vi "LeCroy.Configure Trigger.vi"(5 "Trigger Source":u16(ring) items=["Channel 1", "Channel 2", "Channel 3", "Channel 4", "External", "Line", "Ext", "Ext10"], 7 "Trigger Slope":u16(ring) items=["Rising", "Falling"], 8 "Error In":errorcluster, 10 "Trigger Level":dbl, 11 "LeCroy.Session in":T1) -> (0 "Error Out":errorcluster, 3 "LeCroy.Session out":T1)   [LabVIEW 2018]
uses:
  typedefs/LeCroy.Session.ctl
  <instrlib>/LeCroy Wave Series/Public/Configure/Configure Edge Trigger.vi
  <instrlib>/LeCroy Wave Series/LeCroy Wave Series.lvlib
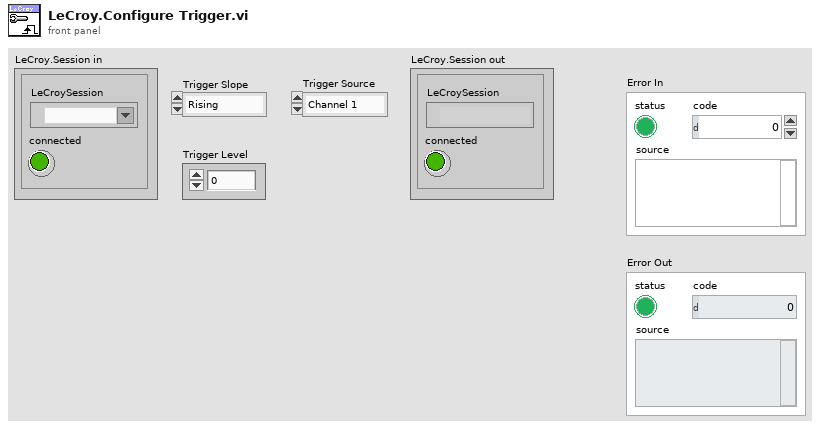
[diagram p1: front panel]
types:
  T1 = typedef "LeCroy.Session.ctl" = cluster{"LeCroySession":refnum<visa-resource-name>, "connected":bool}
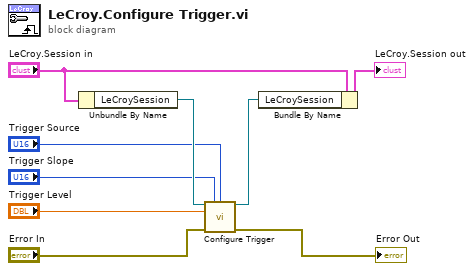
[diagram p0: block diagram]
diagram:
  n1 = Unbundle By Name("LeCroy.Session in") -> ("LeCroySession"=w9:refnum<visa-resource-name>)
  n2 = call-poly <instrlib>:"Configure Trigger.vi"("VISA resource name"=w9, "Trigger Slope (0: Rising)"="Trigger Slope", "Trigger Source (0: Channel 1)"="Trigger Source", "Trigger Level (0.0 V)"="Trigger Level", "error in (no error)"="Error In") -> ("VISA resource name out"=w8:refnum<visa-resource-name>, "error out"=→"Error Out":errorcluster)  [unwired: 9 in]
  n3 = Bundle By Name(cluster="LeCroy.Session in", "LeCroySession"=w8) -> (→"LeCroy.Session out":T1)
